vi "Joystick2RobotMotorCommands.vi"(9 "Joystick R":dbl, 10 "Joystick Y":dbl, 11 "Joystick X":dbl) -> (3 "Robot Motion Commands":T1)   [LabVIEW 2019]
uses:
  Controls/Robot Pivot Motion Commands.ctl
  Controls/Pivot Motor Commands.ctl
  Controls/Robot Drive Mode.ctl
  <vilib>/Rock Robotics/Network Tables/NT Write Numeric Array.vi
panel:
  out "D":dbl
  out "C":dbl
  out "B":dbl
  out "A":dbl
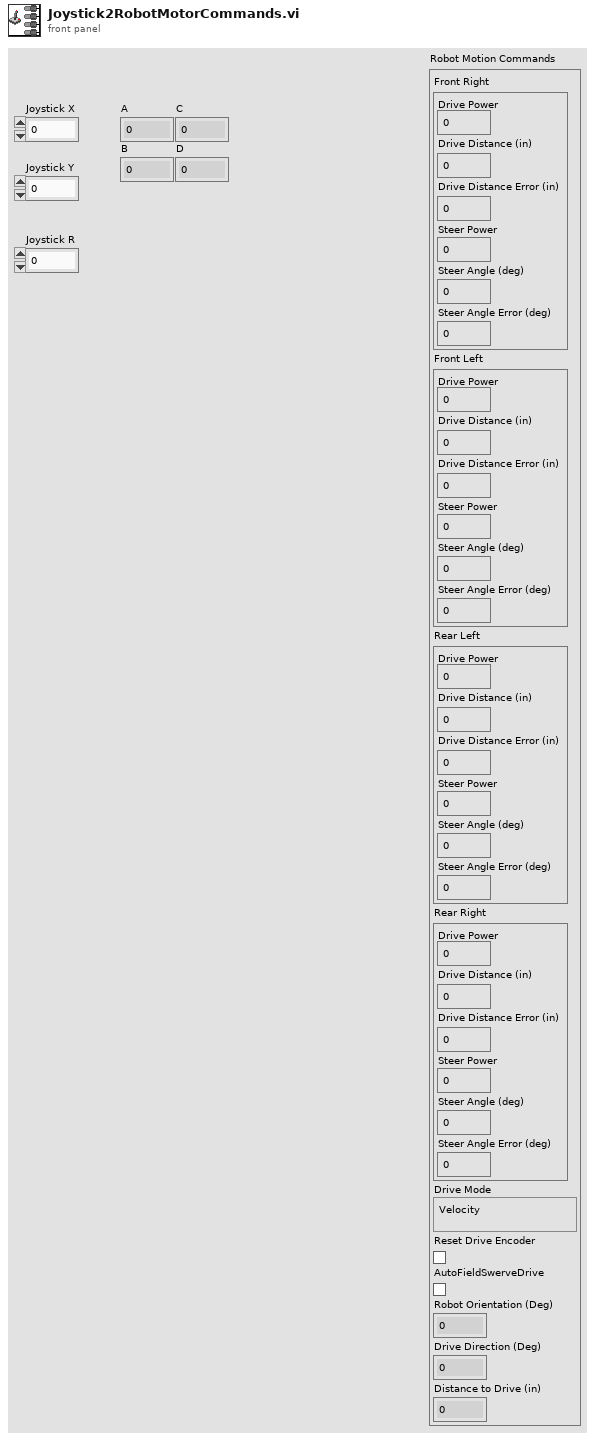
[diagram p1: front panel]
types:
  T1 = typedef "Robot Pivot Motion Commands.ctl" = cluster{"Front Right":T2, "Front Left":T2, "Rear Left":T2, "Rear Right":T2, "Drive Mode":T3, "Reset Drive Encoder":bool, "AutoFieldSwerveDrive":bool, "Robot Orientation (Deg)":dbl, "Drive Direction (Deg)":dbl, "Distance to Drive (in)":dbl}
  T2 = typedef "Pivot Motor Commands.ctl" = cluster{"Drive Power":dbl, "Drive Distance (in)":dbl, "Drive Distance Error (in)":dbl, "Steer Power":dbl, "Steer Angle (deg)":dbl, "Steer Angle Error (deg)":dbl}
  T3 = typedef "Robot Drive Mode.ctl" = enum16{"Velocity", "Distance"}
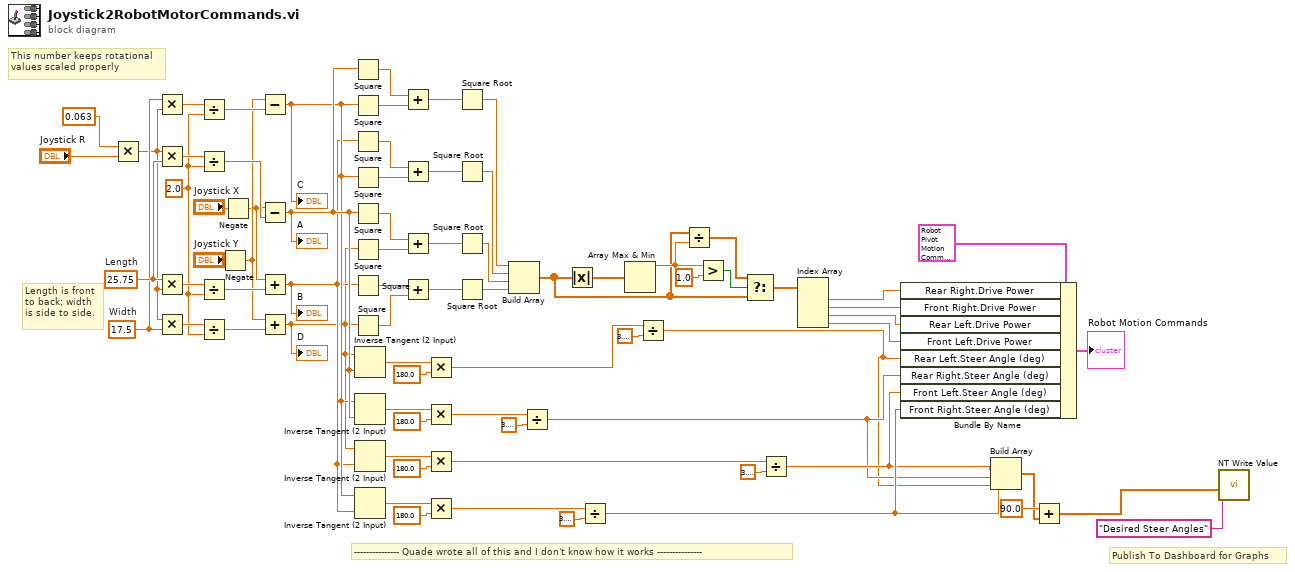
[diagram p0: block diagram]
diagram:
  w34 = 2.0
  w35 = 17.5  # Width
  w72 = 25.75  # Length
  # "Publish To Dashboard for Graphs"
  # "--------------- Quade wrote all of this and I don't know how it works ---------------"
  # "This number keeps rotational\nvalues scaled properly"
  # "Length is front\nto back; width\nis side to side."
  n1 = Multiply(x=0.063, y="Joystick R") -> (x*y=w29:dbl)
  n2 = Multiply(x=w35, y=w29) -> (x*y=w69:dbl)
  n3 = Multiply(x=w29, y=w72) -> (x*y=w75:dbl)
  n4 = Multiply(x=w72, y=w29) -> (x*y=w71:dbl)
  n5 = Multiply(x=w29, y=w35) -> (x*y=w66:dbl)
  n6 = Divide(x=w69, y=w34) -> (x/y=w68:dbl)
  n7 = Divide(x=w75, y=w34) -> (x/y=w74:dbl)
  n8 = Divide(x=w71, y=w34) -> (x/y=w70:dbl)
  n9 = Divide(x=w66, y=w34) -> (x/y=w65:dbl)
  n10 = Negate(x="Joystick Y") -> (-x=w10:dbl)
  n11 = Negate(x="Joystick X") -> (-x=w9:dbl)
  n12 = Subtract(x=w10, y=w68) -> (x-y=w32:dbl)
  "C" <- w32
  n13 = Subtract(x=w9, y=w74) -> (x-y=w33:dbl)
  "A" <- w33
  n14 = Add(x=w9, y=w70) -> (x+y=w31:dbl)
  "B" <- w31
  n15 = Add(x=w10, y=w65) -> (x+y=w30:dbl)
  "D" <- w30
  n16 = Square(x=w33) -> (x^2=w39:dbl)
  n17 = Square(x=w32) -> (x^2=w38:dbl)
  n18 = Square(x=w31) -> (x^2=w60:dbl)
  n19 = Square(x=w32) -> (x^2=w59:dbl)
  n20 = Square(x=w33) -> (x^2=w46:dbl)
  n21 = Square(x=w30) -> (x^2=w45:dbl)
  n22 = Square(x=w31) -> (x^2=w53:dbl)
  n23 = Square(x=w30) -> (x^2=w52:dbl)
  n24 = Inverse Tangent (2 Input)(1:w33, 2:w30) -> (0:w50:dbl)
  n25 = Inverse Tangent (2 Input)(1:w33, 2:w32) -> (0:w43:dbl)
  n26 = Inverse Tangent (2 Input)(1:w31, 2:w30) -> (0:w57:dbl)
  n27 = Inverse Tangent (2 Input)(1:w31, 2:w32) -> (0:w64:dbl)
  n28 = Add(x=w39, y=w38) -> (x+y=w37:dbl)
  n29 = Add(x=w60, y=w59) -> (x+y=w58:dbl)
  n30 = Add(x=w46, y=w45) -> (x+y=w44:dbl)
  n31 = Add(x=w53, y=w52) -> (x+y=w51:dbl)
  n32 = Multiply(x=w50, y=180.0) -> (x*y=w47:dbl)
  n33 = Multiply(x=w43, y=180.0) -> (x*y=w41:dbl)
  n34 = Multiply(x=w57, y=180.0) -> (x*y=w54:dbl)
  n35 = Multiply(x=w64, y=180.0) -> (x*y=w61:dbl)
  n36 = Square Root(x=w37) -> (sqrt(x)=w28:dbl)
  n37 = Square Root(x=w58) -> (sqrt(x)=w27:dbl)
  n38 = Square Root(x=w44) -> (sqrt(x)=w26:dbl)
  n39 = Square Root(x=w51) -> (sqrt(x)=w25:dbl)
  n40 = Build Array(w28, w27, w26, w25) -> (w19:dbl[])
  n41 = Divide(x=w41, y=3.141592653589793) -> (x/y=w5:dbl)
  n42 = Absolute Value(x=w19) -> (abs(x)=w24:dbl[])
  n43 = Divide(x=w61, y=3.141592653589793) -> (x/y=w7:dbl)
  n44 = Array Max & Min(array=w24) -> (max value=w21:dbl)  [unwired: 3 out]
  n45 = Divide(x=w47, y=3.141592653589793) -> (x/y=w4:dbl)
  n46 = Divide(x=w19, y=w21) -> (x/y=w20:dbl[])
  n47 = Greater?(x=w21, y=1.0) -> (0:w22:bool)
  n48 = Select(t=w20, s=w22, f=w19) -> (s? t:f=w18:dbl[])
  n49 = Divide(x=w54, y=3.141592653589793) -> (x/y=w6:dbl)
  n50 = Index Array(array=w18) -> (element #1=w17:dbl, element #2=w16:dbl, element #3=w15:dbl, element #4=w14:dbl)  [unwired: 4 in]
  n51 = Bundle By Name(cluster=T1 {"Front Right"={"Drive Power"=0.0, "Drive Distance (in)"=0.0, "Drive Distance Error (in)"=0.0, "Steer Power"=0.0, "Steer Angle (deg)"=0.0, "Steer Angle Error (deg)"=0.0}, "Front Left"={"Drive Power"=0.0, "Drive Distance (in)"=0.0, "Drive Distance Error (in)"=0.0, "Steer Power"=0.0, "Steer Angle (deg)"=0.0, "Steer Angle Error (deg)"=0.0}, "Rear Left"={"Drive Power"=0.0, "Drive Distance (in)"=0.0, "Drive Distance Error (in)"=0.0, "Steer Power"=0.0, "Steer Angle (deg)"=0.0, "Steer Angle Error (deg)"=0.0}, "Rear Right"={"Drive Power"=0.0, "Drive Distance (in)"=0.0, "Drive Distance Error (in)"=0.0, "Steer Power"=0.0, "Steer Angle (deg)"=0.0, "Steer Angle Error (deg)"=0.0}, "Drive Mode"=enum."Velocity", "Reset Drive Encoder"=FALSE, "AutoFieldSwerveDrive"=FALSE, "Robot Orientation (Deg)"=0.0, "Drive Direction (Deg)"=0.0, "Distance to Drive (in)"=0.0} ("Robot Motion Commands 2"), "Rear Right.Drive Power"=w17, "Front Right.Drive Power"=w16, "Rear Left.Drive Power"=w15, "Front Left.Drive Power"=w14, "Rear Left.Steer Angle (deg)"=w4, "Rear Right.Steer Angle (deg)"=w5, "Front Left.Steer Angle (deg)"=w6, "Front Right.Steer Angle (deg)"=w7) -> (→"Robot Motion Commands":T1)
  n52 = Build Array(w7, w6, w5, w4) -> (w2:dbl[])
  n53 = Add(x=90.0, y=w2) -> (x+y=w1:dbl[])
  n54 = call-poly <vilib>:"NT Write Value.vi"("Numeric Array"=w1, "Name"="Desired Steer Angles") -> ()  [unwired: 9 in, 1 out]
